vi "FABR-Initialize.vi"(0 "Params":T3={"Stimulus"={"Destination"="", "Rep rate (/sec)"=30.0, "Alternate Polarity"=FALSE, "Duration (ms)"=0.0, "Ramp (ms)"=16.0, "Fs (Hz)"=5.0, "Frame size (s)"=0.0}, "Sequence"={"Freq"={"Start (kHz)"=20.0, "Stop (kHz)"=80.0, "Step (oct)"=5.0, "Skip (oct)"=0.0}, "Level"={"Start (dB)"=20, "Stop (dB)"=80, "Step (dB)"=5}, "Order"=enum."Interleaved"}, "Response"={"Gain"=1.0, "Averages"=0, "Window (ms)"=0.0, "Fs (Hz)"=25000.0}, "Reject"=0.0} {"Sequence"."Level"."Start (dB)" step=5; "Sequence"."Freq"."Start (kHz)" step=5.0; "Response"."Window (ms)" format="%.2f"}, 5 "Path":path) -> (4 "Runtime":T8, 8 "SCL":cluster{T1[]}[](array[cluster]), 13 "Analysis":T2, 15 "error out":errorcluster)   [LabVIEW 2020]
uses:
  Typedefs/FABR-Runtime Data.ctl
  Typedefs/FABR-Stimulus Ticket.ctl
  Typedefs/FABR-Parameters.ctl
  Typedefs/FABR-Stimulus.ctl
  Typedefs/FABR-Sequence.ctl
  Typedefs/FABR-Order.ctl
  Typedefs/FABR-Response.ctl
  Typedefs/FABR-Analysis State.ctl
  Typedefs/FABR-Stimulus Condition.ctl
panel:
  in  "error in (no error)":errorcluster
  # "Freq X Level X Time"
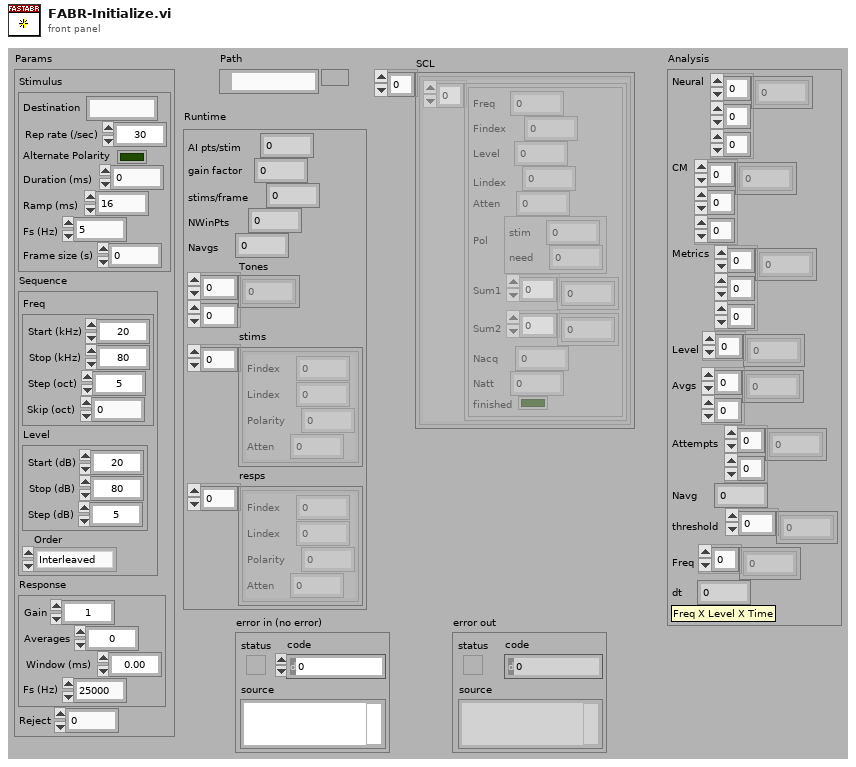
[diagram p1: front panel]
types:
  T1 = typedef "FABR-Stimulus Condition.ctl" = cluster{"Freq":dbl, "Findex":i32, "Level":dbl, "Lindex":i32, "Atten":dbl, "Pol":cluster{"stim":i32, "need":i32}, "Sum1":dbl[], "Sum2":dbl[], "Nacq":i32, "Natt":i32, "finished":bool}
  T2 = typedef "FABR-Analysis State.ctl" = cluster{"Neural":dbl[][][], "CM":dbl[][][], "Metrics":dbl[][][], "Level":dbl[], "Avgs":i32[][], "Attempts":i32[][], "Navg":i32, "threshold":dbl[], "Freq":dbl[], "dt":dbl}
  T3 = typedef "FABR-Parameters.ctl" = cluster{"Stimulus":T4, "Sequence":T5, "Response":T7, "Reject":dbl}
  T4 = typedef "FABR-Stimulus.ctl" = cluster{"Destination":string, "Rep rate (/sec)":dbl, "Alternate Polarity":bool, "Duration (ms)":dbl, "Ramp (ms)":dbl, "Fs (Hz)":dbl, "Frame size (s)":dbl}
  T5 = typedef "FABR-Sequence.ctl" = cluster{"Freq":cluster{"Start (kHz)":dbl, "Stop (kHz)":dbl, "Step (oct)":dbl, "Skip (oct)":dbl}, "Level":cluster{"Start (dB)":i32, "Stop (dB)":i32, "Step (dB)":i32}, "Order":T6}
  T6 = typedef "FABR-Order.ctl" = enum16{"Interleaved"}
  T7 = typedef "FABR-Response.ctl" = cluster{"Gain":dbl, "Averages":i32, "Window (ms)":sgl, "Fs (Hz)":dbl}
  T8 = typedef "FABR-Runtime Data.ctl" = cluster{"AI pts/stim":i32, "gain factor":dbl, "stims/frame":i32, "NWinPts":i32, "Navgs":i32, "Tones":dbl[][], "stims":T9[], "resps":T9[]}
  T9 = typedef "FABR-Stimulus Ticket.ctl" = cluster{"Findex":i32, "Lindex":i32, "Polarity":i32, "Atten":dbl}
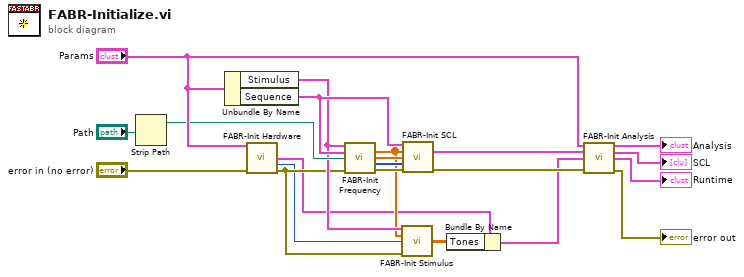
[diagram p0: block diagram]
diagram:
  n1 = Strip Path(path="Path") -> (stripped path=w16:path)  [unwired: 1 out]
  n2 = Unbundle By Name("Params") -> ("Stimulus"=w11:T4, "Sequence"=w14:T5)
  n3 = call "FABR-Init Hardware.vi"("Params"="Params", "error in (no error)"="error in (no error)") -> ("Runtime"=w6:T8, "AO npts"=w8:i32, "error out"=w9:errorcluster)  [unwired: 11 in]
  n4 = call "FABR-Init Frequency.vi"("Stimulus"=w11, "Sequence"=w14, "Data folder"=w16, "error in (no error)"=w9) -> ("Frequency (kHz)"=w10:dbl[], "Ceilings"=w13:dbl[], "Order"=w12:i32[], "error out"=w15:errorcluster)  [unwired: 8 in]
  n5 = call "FABR-Init Stimulus.vi"("Stimulus"=w11, "Frequency"=w10, "Npts"=w8, "error in (no error)"=w9) -> ("Tones"=w3:dbl[][])  [unwired: 10 in, 1 out]
  n6 = call "FABR-Init SCL.vi"("Sequence"=w14, "Frequency"=w10, "Ceiling"=w13, "Order"=w12, "error in (no error)"=w15) -> ("SCL"=w2:cluster{T1[]}[], "error out"=w7:errorcluster)  [unwired: 9 in]
  n7 = Bundle By Name(cluster=w6, "Tones"=w3) -> (w4:T8)
  n8 = call "FABR-Init Analysis.vi"("Params"="Params", "SCL in"=w2, "Runtime in"=w4, "error in (no error)"=w7) -> ("Analysis"=→"Analysis":T2, "SCL out"=→"SCL":cluster{T1[]}[], "Runtime out"=→"Runtime":T8, "error out"=→"error out":errorcluster)  [unwired: 8 in]
